vi "Delete from Array of Instrument Addresses.vi"(8 "error in (no error)":errorcluster, 11 "Instrument Finder in":refnum<class "Instrument Finder.lvclass">) -> (0 "error out":errorcluster, 3 "Instrument Finder out":refnum<class "Instrument Finder.lvclass">)   [LabVIEW 2014, in "SetUp VIs.lvlib" / "Instrument Finder.lvclass"]
uses:
  Instrument Finder.lvclass
  <vilib>/ActorFramework/Message Enqueuer/Message Enqueuer.lvclass
panel:
  in  "element":refnum<class "Message Enqueuer.lvclass">
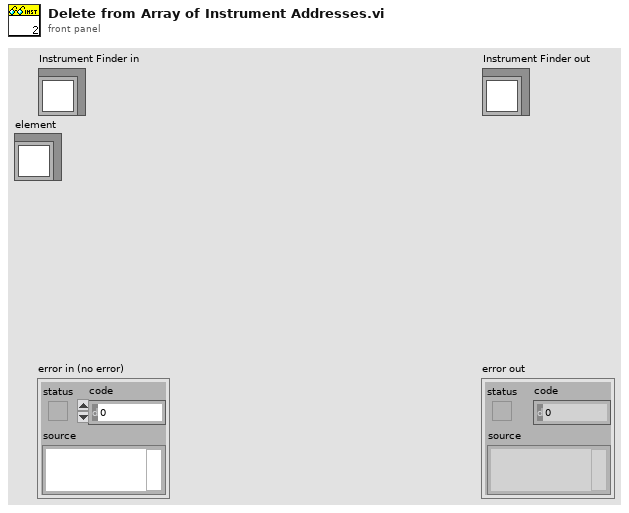
[diagram p1: front panel]
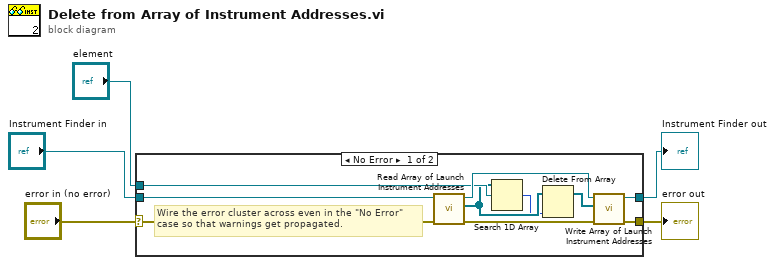
[diagram p0: block diagram]
diagram:
  n1 = case shown="No Error" "error in (no error)" {
    selector: "error in (no error)" -> [w12 w17]
    tunnel: [w6 w17] -> w4
    tunnel: [w13 w16] -> w2
    tunnel: "Instrument Finder in" -> [w15 w16]
    tunnel: "element" -> [w11 _]
    frame No Error {
      # "Wire the error cluster across even in the \"No Error\"\ncase so that warnings get propagated."
      n2 = call-dynamic "Read Array of Launch Instrument Addresses.vi"("error in (no error)"=w12, "Instrument Finder in"=w15) -> ("error out"=w7:errorcluster, "Array of Launch Instrument Addresses"=w10:refnum<class "Message Enqueuer.lvclass">[], "Instrument Finder out"=w14:refnum<class "Instrument Finder.lvclass">)  [unwired: 7 in]
      n3 = Search 1D Array(1D array=w10, element=w11) -> (index of element=w9:i32)  [unwired: 1 in]
      n4 = Delete From Array(array=w10, index=w9) -> (array with subset deleted=w8:refnum<class "Message Enqueuer.lvclass">[])  [unwired: 1 in, 1 out]
      n5 = call-dynamic "Write Array of Launch Instrument Addresses.vi"("error in (no error)"=w7, "Array of Launch Instrument Addresses"=w8, "Instrument Finder in"=w14) -> ("error out"=w6:errorcluster, "Instrument Finder out"=w13:refnum<class "Instrument Finder.lvclass">)  [unwired: 7 in]
    }
    frame Error {
    }
  }
  "error out" <- w4
  "Instrument Finder out" <- w2
